vi "Alimentacion1.vi"(1 "VoltajeDeseado":dbl) -> (0 "Numeric Indicator":dbl)   [LabVIEW 2017]
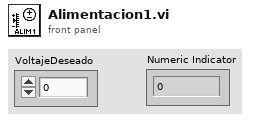
[diagram p1: front panel]
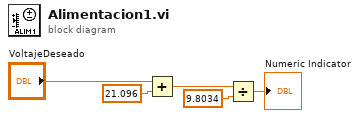
[diagram p0: block diagram]
diagram:
  n1 = Add(x="VoltajeDeseado", y=21.096) -> (x+y=w3:dbl)
  n2 = Divide(x=w3, y=9.8034) -> (x/y=→"Numeric Indicator":dbl)
